vi "Decode frame.vi"(8 "error in (no error)":errorcluster, 11 "frame data":u8[](array[numeric])) -> (0 "error out":errorcluster, 2 "Payload_String":string, 3 "Ethernet Header Cluster":T1 {"Ethertype" format="%.0x"; "VLAN Tag"."VID" format="%.0x"; "VLAN Tag"."TPID" format="%.0x"; "source MAC address"."?" format="%02x"; "source MAC address"."?" format="%02x"; "source MAC address"."?" format="%02x"; "source MAC address"."?" format="%02x"; "source MAC address"."?" format="%02x"; "source MAC address"."?" format="%02x"; "destination MAC address"."?" format="%02x"; "destination MAC address"."?" format="%02x"; "destination MAC address"."?" format="%02x"; "destination MAC address"."?" format="%02x"; "destination MAC address"."?" format="%02x"; "destination MAC address"."?" format="%02x"})   [LabVIEW 2025, in "Automotive Ethernet Bus Monitor UI.lvlib"]
uses:
  Automotive Ethernet Bus Monitor UI.lvlib
  Ethernet Header Cluster.ctl
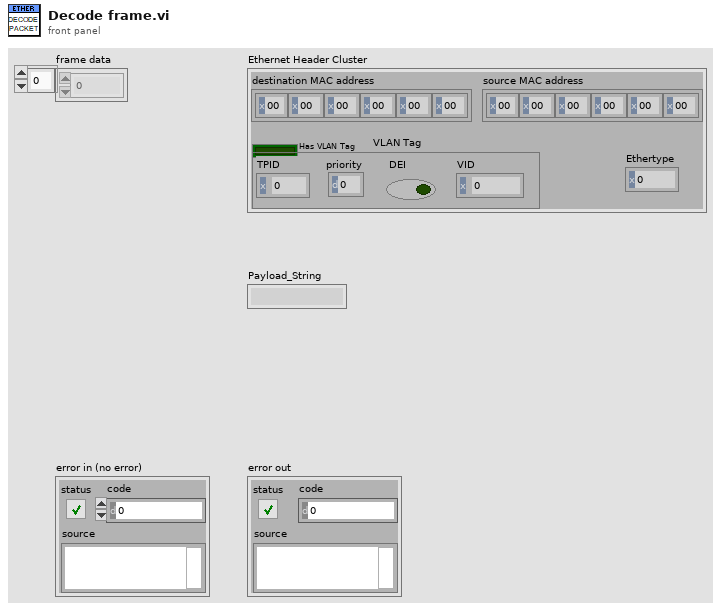
[diagram p1: front panel]
types:
  T1 = typedef "Automotive Ethernet Bus Monitor UI.lvlib/Ethernet Header Cluster.ctl" = cluster{"destination MAC address":cluster{u8, u8, u8, u8, u8, u8}, "source MAC address":cluster{u8, u8, u8, u8, u8, u8}, "Has VLAN Tag":bool, "VLAN Tag":cluster{"TPID":u16, "priority":u8, "DEI":bool, "VID":u16}, "Ethertype":u16}
  T2 = cluster{"destination MAC address":cluster{u8, u8, u8, u8, u8, u8}, "source MAC address":cluster{u8, u8, u8, u8, u8, u8}, "Has VLAN Tag":bool, "VLAN Tag":cluster{"TPID":u16, "priority":u8, "DEI":bool, "VID":u16}, "Ethertype":u16}
  T3 = cluster{"destination MAC address":cluster{u8, u8, u8, u8, u8, u8}, "source MAC address":cluster{u8, u8, u8, u8, u8, u8}, "length / type":u16}
  T4 = cluster{"TPID":u16, "priority":u8, "DEI":bool, "VID":u16}
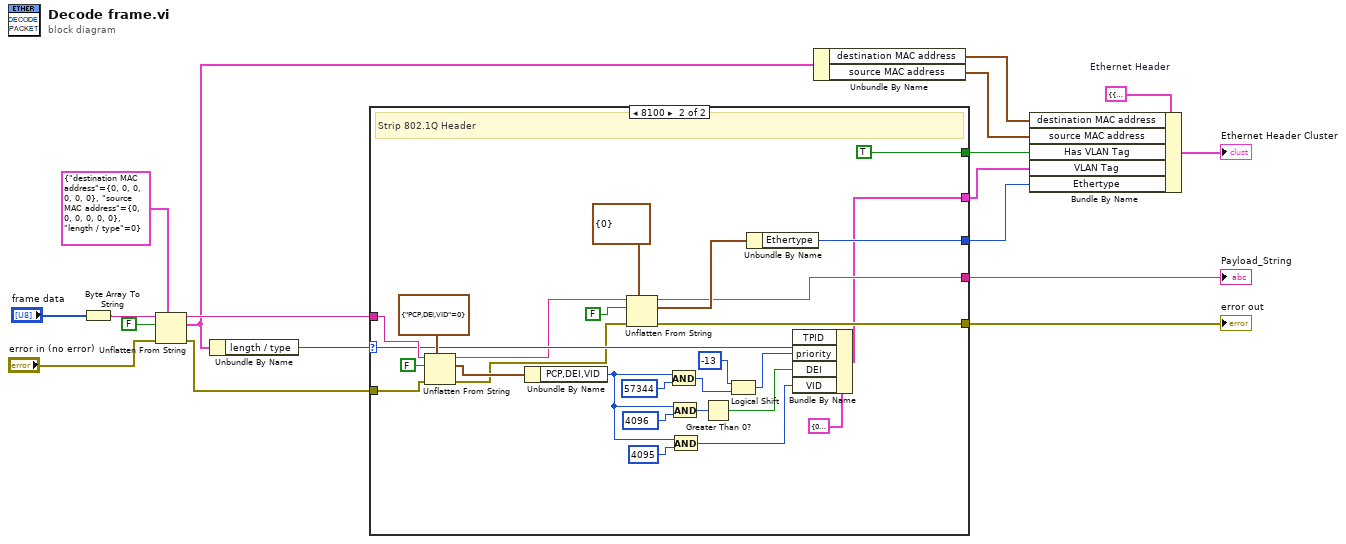
[diagram p0: block diagram]
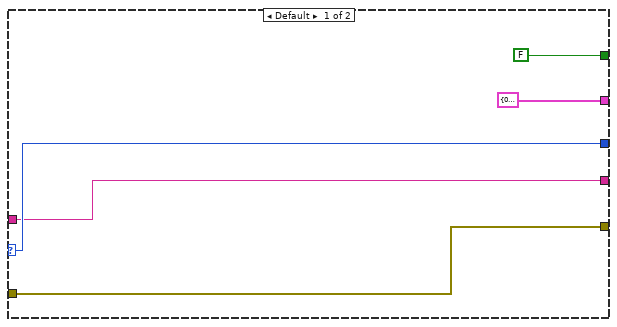
[diagram p2: hidden frame]
diagram:
  w9 = T2 {"destination MAC address"={0, 0, 0, 0, 0, 0}, "source MAC address"={0, 0, 0, 0, 0, 0}, "Has VLAN Tag"=FALSE, "VLAN Tag"={"TPID"=0, "priority"=0, "DEI"=FALSE, "VID"=0}, "Ethertype"=0}  # Ethernet Header
  n1 = Byte Array To String(unsigned byte array="frame data") -> (string=w1:string)
  n2 = Unflatten From String(type=T3 {"destination MAC address"={0, 0, 0, 0, 0, 0}, "source MAC address"={0, 0, 0, 0, 0, 0}, "length / type"=0} ("ethernet header"), binary string=w1, data includes array or string size? (T)=FALSE, error in (no error)="error in (no error)") -> (rest of the binary string=w16:string, value=w14:T3, error out=w11:errorcluster)  [unwired: 1 in]
  n3 = Unbundle By Name(w14) -> ("length / type"=w15:u16)
  n4 = case shown="8100" w15 {
    selector: w15 -> [w23 w37]
    tunnel: w16 -> [w22 w50]
    tunnel: [w23 w31] -> w8
    tunnel: [w22 w30] -> w13
    tunnel: w11 -> [w21 w29]
    tunnel: [w21 w27] -> w10
    tunnel: [T4 {"TPID"=0, "priority"=0, "DEI"=FALSE, "VID"=0} ("802.1Q Header") w26] -> w7
    tunnel: [FALSE ("data includes array or string size? (T)") TRUE ("data includes array or string size? (T)")] -> w6
    frame Default {
    }
    frame 33024 {
      # "Strip 802.1Q Header"
      n5 = Unflatten From String(type=cluster{"PCP,DEI,VID":u16} {"PCP,DEI,VID"=0}, binary string=w50, data includes array or string size? (T)=FALSE, error in (no error)=w29) -> (rest of the binary string=w24:string, value=w47:cluster{"PCP,DEI,VID":u16}, error out=w28:errorcluster)  [unwired: 1 in]
      n6 = Unbundle By Name(w47) -> ("PCP,DEI,VID"=w39:u16)
      n7 = Unflatten From String(type=cluster{"Ethertype":u16} {"Ethertype"=0}, binary string=w24, data includes array or string size? (T)=FALSE, error in (no error)=w28) -> (rest of the binary string=w30:string, value=w34:cluster{"Ethertype":u16}, error out=w27:errorcluster)  [unwired: 1 in]
      n8 = And(x=w39, y=u16 57344) -> (x .and. y?=w33:u16)
      n9 = And(x=w39, y=u16 4096) -> (x .and. y?=w42:u16)
      n10 = And(x=w39, y=u16 4095) -> (x .and. y?=w38:u16)
      n11 = Greater Than 0?(x=w42) -> (x > 0?=w41:bool)
      n12 = Logical Shift(y=i16 -13, x=w33) -> (x << y=w44:u16)
      n13 = Unbundle By Name(w34) -> ("Ethertype"=w31:u16)
      n14 = Bundle By Name(cluster=T4 {"TPID"=0, "priority"=0, "DEI"=FALSE, "VID"=0} ("802.1Q Header"), "TPID"=w37, "priority"=w44, "DEI"=w41, "VID"=w38) -> (w26:T4)
    }
  }
  "Payload_String" <- w13
  "error out" <- w10
  n15 = Unbundle By Name(w14) -> ("destination MAC address"=w5:cluster{u8, u8, u8, u8, u8, u8}, "source MAC address"=w4:cluster{u8, u8, u8, u8, u8, u8})
  n16 = Bundle By Name(cluster=w9, "destination MAC address"=w5, "source MAC address"=w4, "Has VLAN Tag"=w6, "VLAN Tag"=w7, "Ethertype"=w8) -> (→"Ethernet Header Cluster":T2)
